vi "SistemaAireCaliente.vi"() -> ()   [LabVIEW 2010]
uses:
  <vilib>/Platform/TimedLoop/XDataNode/XDataNode.xnode
  <vilib>/Platform/TimedLoop/XDataNode/timing_clust.ctl
  <vilib>/Platform/TimedLoop/XDataNode/nitl_modes.ctl
  <vilib>/Platform/TimedLoop/XDataNode/wakeup.ctl
  <vilib>/Instr/_visa.llb/VISA Configure Serial Port (Instr).vi
  <vilib>/Platform/TimedLoop/XDataNode/XDNodeRunTimeDep.lvlib
panel:
  in  "velocidad":dbl(slide) scale=0.0..40.0
  in  "AUTOMATICO":bool
  in  "Ajuste":dbl(slide) scale=0.0..10.0
  out "TEMP EXTERNA":dynamicdata(graph)
  out "TEMP INTERNA":i32(graph)
  out "Temp Externa":i32
  out "Temp Externa":dbl(slide) scale=20.0..150.0
  out "Temp Interna":dbl(slide) scale=20.0..200.0
  in  "Set- Point\n Temperatura Exterior (C)":u32(slide) scale=0.0..150.0
  in  "Period                :":i64=1000
  in  "Flow control    :":u16(ring) items=["None"=0, "XON/XOFF"=1, "RTS/CTS"=2, "DTR/DSR"=4]
  in  "Stop bits         :":u16(ring)=10 items=["1.0"=10, "1.5"=15, "2.0"=20]
  in  "Paridad            :":u16(ring) items=["None", "Odd", "Even", "Mark", "Space"]
  in  "Data bits          :":u16=8 min=5 max=8 step=1
  in  "VISA resource : name:":refnum<visa-resource-name>="COM1"
  in  "Baud rate         :":u32=9600
  in  "stop":bool
  out "Read buffer":string
  out "Temp Interna":i32
  # "Control de Temperatura"
  # "Configuracion Serial"
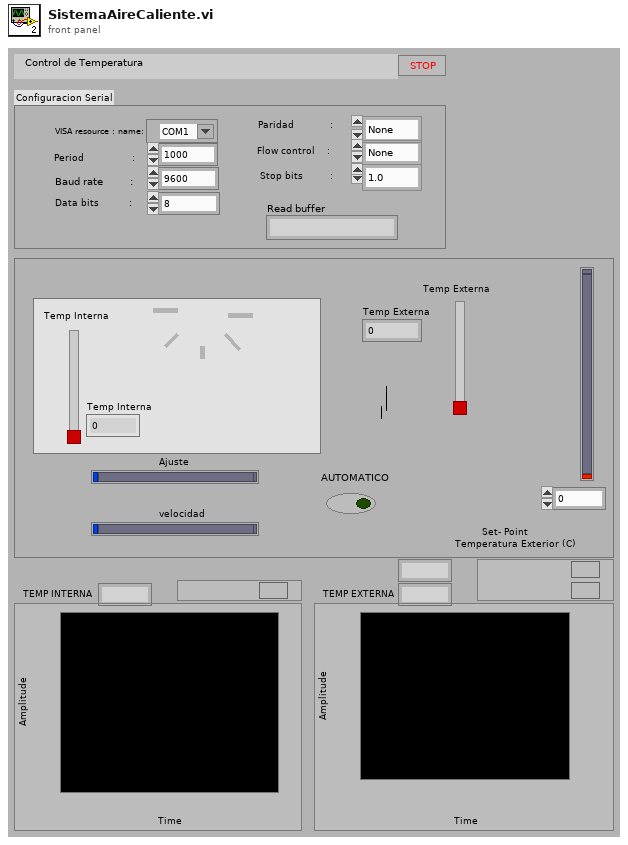
[diagram p1: front panel]
types:
  T1 = typedef "XDNodeRunTimeDep.lvlib/timing_clust.ctl" = cluster{"Expected End [f-1]":u64, "Actual End [f-1]":u64, "Finished Late? [f-1]":bool, "Expected End [i-1]":u64, "Actual End [i-1]":u64, "Finished Late? [i-1]":bool, "Expected Start [i]":u64, "Actual Start [i]":u64, "Expected Start [f]":u64, "Actual Start [f]":u64, "Source Name":string, "Structure Name":string, "Period":i64, "Deadline":i64, "Offset":i64, "Start":i64, "Priority":i32, "Timeout":i32, "Mode":T2, "Wakeup Reason":T3, "Error":errorcluster, "Source Type":string, "Secondary Source Type":string, "Global End Time":u64, "Global Start Time":u64, "Frame Duration":u64, "Iteration Duration":u64, "Assigned CPU":i32, "I/O Scan Engine Mode":u32}
  T2 = typedef "XDNodeRunTimeDep.lvlib/nitl_modes.ctl" = enum32{"No Change", "Process missed periods, maintain original phase", "Discard missed periods, maintain original phase", "Process missed periods, ignore original phase", "Discard missed periods, ignore original phase"}
  T3 = typedef "XDNodeRunTimeDep.lvlib/wakeup.ctl" = enum32{"Normal", "Aborted", "Asynchronous wakeup", "Timing source error", "Timed loop error", "Timeout"}
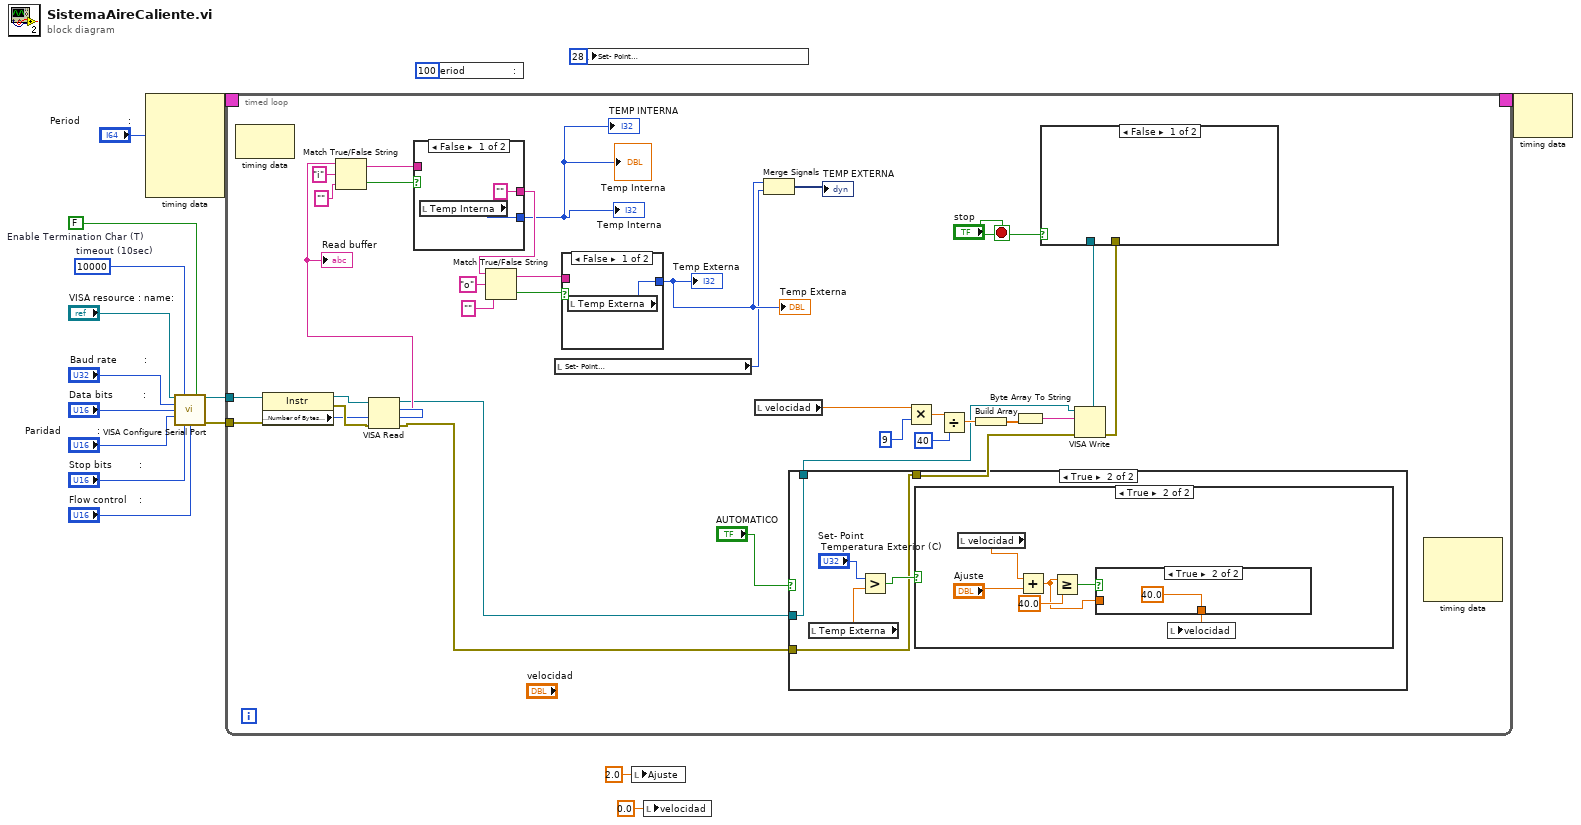
[diagram p0: block diagram]
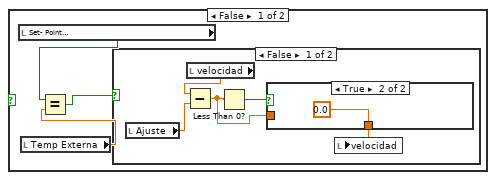
[diagram p3: hidden frame]
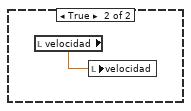
[diagram p5: hidden frame]
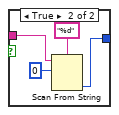
[diagram p7: hidden frame]
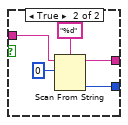
[diagram p8: hidden frame]
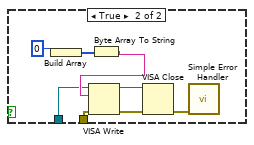
[diagram p9: hidden frame]
diagram:
  w11 = FALSE  # Enable Termination Char (T)
  w12 = u32 10000  # timeout (10sec)
  n1 = node-c288("Period                :") -> (w17:T1)  [unwired: 4 in]
  n2 = call-poly "VISA Configure Serial Port"("VISA resource name"="VISA resource : name:", "timeout (10sec)"=w12, "Enable Termination\nChar (T)"=w11, "baud rate (9600)"="Baud rate         :", "data bits (8)"="Data bits          :", "parity (0:none)"="Paridad            :", "stop bits (10: 1 bit)"="Stop bits         :", "flow control (0:none)"="Flow control    :") -> ("VISA resource name out"=w7:refnum<visa-resource-name>, "error out"=w6:errorcluster)  [unwired: 6 in]
  n3 = timed-loop {
    timing: w17 -> [_]
    timing-out: [_] -> w16
    tunnel: w7 -> [w42]
    tunnel: w6 -> [w41]
    stop <- "stop" stop-if-true
    n4 = node-c288() -> ()  [unwired: 1 in, 1 out]
    n5 = property class="Instr"(reference=w42, error in=w41) -> (reference out=w43:refnum<visa-resource-name>, error out=w51:errorcluster, "Serial Settings:Number of Bytes at Serial Port"=w50:u32)
    n6 = VISA Read(VISA resource name=w43, byte count=w50, error in (no error)=w51) -> (VISA resource name out=w33:refnum<visa-resource-name>, read buffer=w48:string, error out=w32:errorcluster)  [unwired: 1 out]
    "Read buffer" <- w48
    n7 = Match True/False String(2:"" ("false string"), 3:"i" ("true string"), 4:w48) -> (0:w46:bool, 1:w45:string)
    n8 = case shown="False" w46 {
      tunnel: w45 -> [_ w87]
      tunnel: ["" w86] -> w36
      tunnel: [w84 w85] -> w35
      frame False {
        n9 = local read "Temp Interna"() -> (w84:i32)
      }
      frame True {
        n10 = Scan From String(format string="%d", input string=w87, initial scan location=u32 0) -> (remaining string=w86:string, output 1=w85:i32)  [unwired: 2 in, 2 out]
      }
    }
    "Temp Interna" <- w35
    "Temp Interna" <- w35
    "TEMP INTERNA" <- w35
    n11 = Match True/False String(2:"" ("false string"), 3:"o" ("true string"), 4:w36) -> (0:w38:bool, 1:w39:string)
    n12 = local read "Set- Point\n Temperatura Exterior (C)"() -> (w18:u32)
    n13 = case shown="False" w38 {
      tunnel: w39 -> [_ w80]
      tunnel: [w78 w79] -> w19
      frame False {
        n14 = local read "Temp Externa"() -> (w78:i32)
      }
      frame True {
        n15 = Scan From String(format string="%d", input string=w80, initial scan location=u32 0) -> (output 1=w79:i32)  [unwired: 2 in, 3 out]
      }
    }
    "Temp Externa" <- w19
    "Temp Externa" <- w19
    n16 = local read "velocidad"() -> (w25:dbl)
    n17 = Merge Signals(w19, w18) -> (→"TEMP EXTERNA":dynamicdata)
    n18 = case shown="True" "AUTOMATICO" {
      tunnel: w33 -> [w53 w55]
      tunnel: w32 -> [w52 w54]
      tunnel: [w53 w55] -> w24
      tunnel: [w52 w54] -> w23
      frame False {
      }
      frame True {
        n19 = local read "Temp Externa"() -> (w57:dbl)
        n20 = Greater?(x="Set- Point\n Temperatura Exterior (C)", y=w57) -> (0:w56:bool)
        n21 = case shown="True" w56 {
          frame False {
            n22 = local read "Set- Point\n Temperatura Exterior (C)"() -> (w59:u32)
            n23 = local read "Temp Externa"() -> (w61:dbl)
            n24 = Equal?(x=w59, y=w61) -> (x = y?=w60:bool)
            n25 = case shown="False" w60 {
              frame False {
                n26 = local read "Ajuste"() -> (w63:dbl)
                n27 = local read "velocidad"() -> (w66:dbl)
                n28 = Subtract(x=w66, y=w63) -> (x-y=w62:dbl)
                n29 = Less Than 0?(x=w62) -> (x < 0?=w65:bool)
                n30 = case shown="True" w65 {
                  tunnel: [w67 0.0 ("y")] -> w64
                  tunnel: w62 -> [w67 _]
                  frame False {
                  }
                  frame True {
                  }
                }
                n31 = local write "velocidad"(w64) -> ()
              }
              frame True {
                n32 = local read "velocidad"() -> (w69:dbl)
                n33 = local write "velocidad"(w69) -> ()
              }
            }
          }
          frame True {
            n34 = local read "velocidad"() -> (w75:dbl)
            n35 = Add(x=w75, y="Ajuste") -> (x+y=w70:dbl)
            n36 = Greater Or Equal?(x=w70, y=40.0) -> (x >= y?=w72:bool)
            n37 = case shown="True" w72 {
              tunnel: [w76 40.0 ("y")] -> w71
              tunnel: w70 -> [w76 _]
              frame False {
              }
              frame True {
              }
            }
            n38 = local write "velocidad"(w71) -> ()
          }
        }
      }
    }
    n39 = Multiply(x=w25, y=u8 9) -> (x*y=w28:dbl)
    n40 = Divide(x=w28, y=u8 40) -> (x/y=w26:dbl)
    n41 = Build Array(w26) -> (w31:dbl[])
    n42 = Byte Array To String(unsigned byte array=w31) -> (string=w30:string)
    n43 = VISA Write(VISA resource name=w24, write buffer=w30, error in (no error)=w23) -> (VISA resource name out=w22:refnum<visa-resource-name>, error out=w21:errorcluster)  [unwired: 1 out]
    n44 = case shown="False" "stop" {
      tunnel: w22 -> [_ w91]
      tunnel: w21 -> [_ w90]
      frame False {
      }
      frame True {
        n45 = Build Array(0 ("number")) -> (w92:i32[])
        n46 = Byte Array To String(unsigned byte array=w92) -> (string=w94:string)
        n47 = VISA Write(VISA resource name=w91, write buffer=w94, error in (no error)=w90) -> (VISA resource name out=w96:refnum<visa-resource-name>, error out=w95:errorcluster)  [unwired: 1 out]
        n48 = VISA Close(VISA resource name=w96, error in (no error)=w95) -> (error out=w97:errorcluster)
        n49 = call <vilib>:"Simple Error Handler.vi"("error in (no error)"=w97) -> ()  [unwired: 4 in, 5 out]
      }
    }
    n50 = node-c288() -> ()  [unwired: 3 in, 1 out]
  }
  n51 = local write "Period                :"(i64 100 ("Period")) -> ()
  n52 = local write "Set- Point\n Temperatura Exterior (C)"(u8 28 ("Set- Point\n Temperatura Exterior (C)")) -> ()
  n53 = local write "Ajuste"(2.0 ("Ajuste")) -> ()
  n54 = local write "velocidad"(0.0 ("velocidad")) -> ()
  n55 = node-c288(w16) -> ()  [unwired: 1 out]
